vi "Get Force Accuracy Test Settings.vi"(11 "Model in":refnum<class "Model.lvclass">) -> (2 "Force Accuracy Test Settings":T1 {"Sample Time (s)" format="%.4f"; "Process Time (s)" format="%.4f"; "Max Moment (NM)" format="%.4f"; "Max Force Error (N)" format="%.4f"}, 3 "Model out":refnum<class "Model.lvclass">)   [LabVIEW 2016]
uses:
  Model.lvclass
  Typedefs/ForceAccuracyTestSettings.ctl
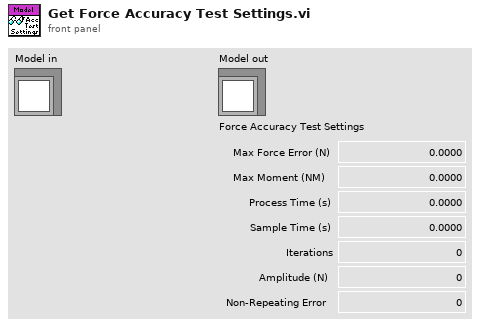
[diagram p1: front panel]
types:
  T1 = typedef "ForceAccuracyTestSettings.ctl" = cluster{"Max Force Error (N)":dbl, "Max Moment (NM)":dbl, "Process Time (s)":dbl, "Sample Time (s)":dbl, "Iterations":i32, "Amplitude (N)":dbl, "Non-Repeating Error":dbl}
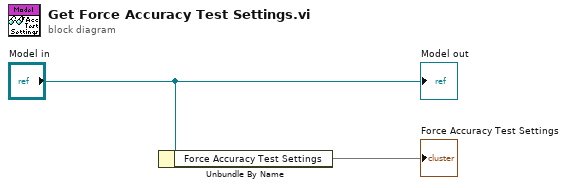
[diagram p0: block diagram]
diagram:
  n1 = Unbundle By Name("Model in") -> ("Force Accuracy Test Settings"=→"Force Accuracy Test Settings")
  "Model out" <- "Model in"
